vi "RichToFlatni_measurementlink_measurement_v2_Output.vi"(5 "OutputClusterType":T1, 11 "InputCluster":T4) -> (3 "OutputCluster":T1)   [LabVIEW 2021, in "Measurement Service Client.lvlib"]
uses:
  Measurement Service Client.lvlib
  ni_measurementlink_measurement_v2_Output_AnnotationsEntry_Flat.ctl
  google_protobuf_Field_Kind.ctl
  ni_measurementlink_measurement_v2_Output_Flat.ctl
  ni_measurementlink_measurement_v2_Output_AnnotationsEntry.ctl
  ni_measurementlink_measurement_v2_Output.ctl
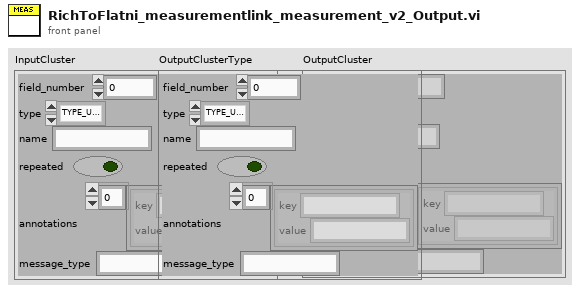
[diagram p1: front panel]
types:
  T1 = typedef "Measurement Service Client.lvlib/ni_measurementlink_measurement_v2_Output_Flat.ctl" = cluster{"field_number":i32, "type":T2, "name":string, "repeated":bool, "annotations":T3[], "message_type":string}
  T2 = typedef "Measurement Service Client.lvlib/google_protobuf_Field_Kind.ctl" = enum32{"TYPE_UNKNOWN", "TYPE_DOUBLE", "TYPE_FLOAT", "TYPE_INT64", "TYPE_UINT64", "TYPE_INT32", "TYPE_FIXED64", "TYPE_FIXED32", "TYPE_BOOL", "TYPE_STRING", "TYPE_GROUP", "TYPE_MESSAGE", "TYPE_BYTES", "TYPE_UINT32", "TYPE_ENUM", "TYPE_SFIXED32", "TYPE_SFIXED64", "TYPE_SINT32", "TYPE_SINT64"}
  T3 = typedef "Measurement Service Client.lvlib/ni_measurementlink_measurement_v2_Output_AnnotationsEntry_Flat.ctl" = cluster{"key":string, "value":string}
  T4 = typedef "Measurement Service Client.lvlib/ni_measurementlink_measurement_v2_Output.ctl" = cluster{"field_number":i32, "type":T2, "name":string, "repeated":bool, "annotations":T5[], "message_type":string}
  T5 = typedef "Measurement Service Client.lvlib/ni_measurementlink_measurement_v2_Output_AnnotationsEntry.ctl" = cluster{"key":string, "value":string}
  T6 = typedef "ni.measurementlink.measurement.v2.api.lvlib/Measurement Service Client.lvlib/ni_measurementlink_measurement_v2_Output_AnnotationsEntry_Flat.ctl" = cluster{"key":string, "value":string}
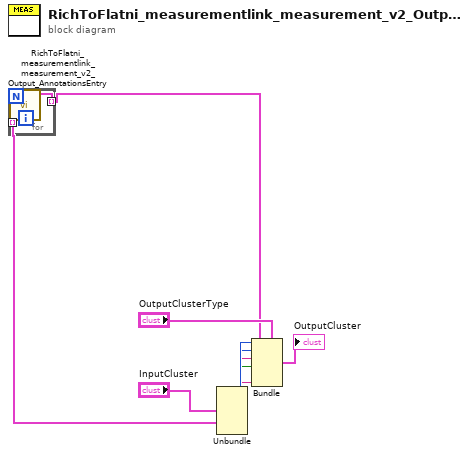
[diagram p0: block diagram]
diagram:
  n1 = Unbundle "Unbundle"("InputCluster") -> ("field_number"=w7:i32, "type"=w6:T2, "name"=w5:string, "repeated"=w4:bool, "annotations"=w3:T5[], "message_type"=w1:string)
  n2 = for {
    tunnel: w3 -> [w12] mode=indexing
    tunnel: [w11] -> w2 mode=indexing
    n3 = call "RichToFlatni_measurementlink_measurement_v2_Output_AnnotationsEntry.vi"("InputCluster"=w12) -> ("OutputCluster"=w11:T6)  [unwired: 10 in]
  }
  n4 = Bundle "Bundle"(cluster="OutputClusterType", "field_number"=w7, "type"=w6, "name"=w5, "repeated"=w4, "annotations"=w2, "message_type"=w1) -> (→"OutputCluster":T1)
